vi "ExperimentProgramUI.vi"() -> ()   [LabVIEW 2011]
uses:
  Motors/MotorAxisEnum.ctl
  Motors/MotorPosType.ctl
  Typedefs/XYf.ctl
  Motors/MotorPosFlagsType.ctl
  Typedefs/MeasureConfigOutputMode.ctl
  Typedefs/CmdEnum_UserInterfaceCmd.ctl
  GlobalVariables.vi
panel:
  in  "Run sections util":bool
  in  "Run experiment":bool
  in  "Which motors should the script control?":T1={"Magnet Z"=TRUE, "Magnet rotation"=TRUE, "Camera"={"X"=FALSE, "Y"=FALSE}, "Piezo XY"={"X"=FALSE, "Y"=FALSE}, "Piezo Z"=FALSE, "Coil XY"={"X"=FALSE, "Y"=FALSE}}
  in  "Program.Motor Axis accuracy conditions":T2
  out "Simulated positions":T2[](array[typedef])
  in  "Axis to show in graph":T4[](array[typedef])=[enum."magrot", enum."magrot", enum."magpos"]
  out "Positions according to program":dbl[][](graph)
  in  "Tab Control 2":enum32{"Script", "Paths & Settings"}(tab)
  in  "Test run without experiment":bool
  in  "Script":string="% Initial position\n%move magpos 20; move magrot 0;\n%wait\n\n% Program\n%move magrot 1000 speed 100; wait;\n%move magrot 50 speed 10;\n%move magpos 10 speed 2;wait\n"
  in  "Simulate script":bool
  in  "Save script":bool
  in  "Load script":bool
  in  "Write interval [frames]":i32
  in  "Experiment base path":path
  in  "Experiment name":string
  out "Traces will end up here:":path
  in  "Output mode":T5=enum."Track"
  in  "Image output path":string
  in  "Trace output path":string
  in  "Max frames in memory":i32
  in  "Save traces as binary":bool
  in  "stop":bool
  # "Axis names:\nmagrot:   Magnet rotation\nmagpos:   Magnet Z (vertical) position\npx, py, pz:   Piezo stage\ncamx, camy: Camera motorized stage"
  # "Instructions:\nmove <axis> <position>;\nMove axis to position at current speed\nmove <axis> <position> speed <speed>;\nMove axis to position at specified speed (units/s)\nidle <seconds>;\nDo nothing for specified time\nsection <optional name>;\nStore current framenumber in section file\nstop;\nStop experiment"
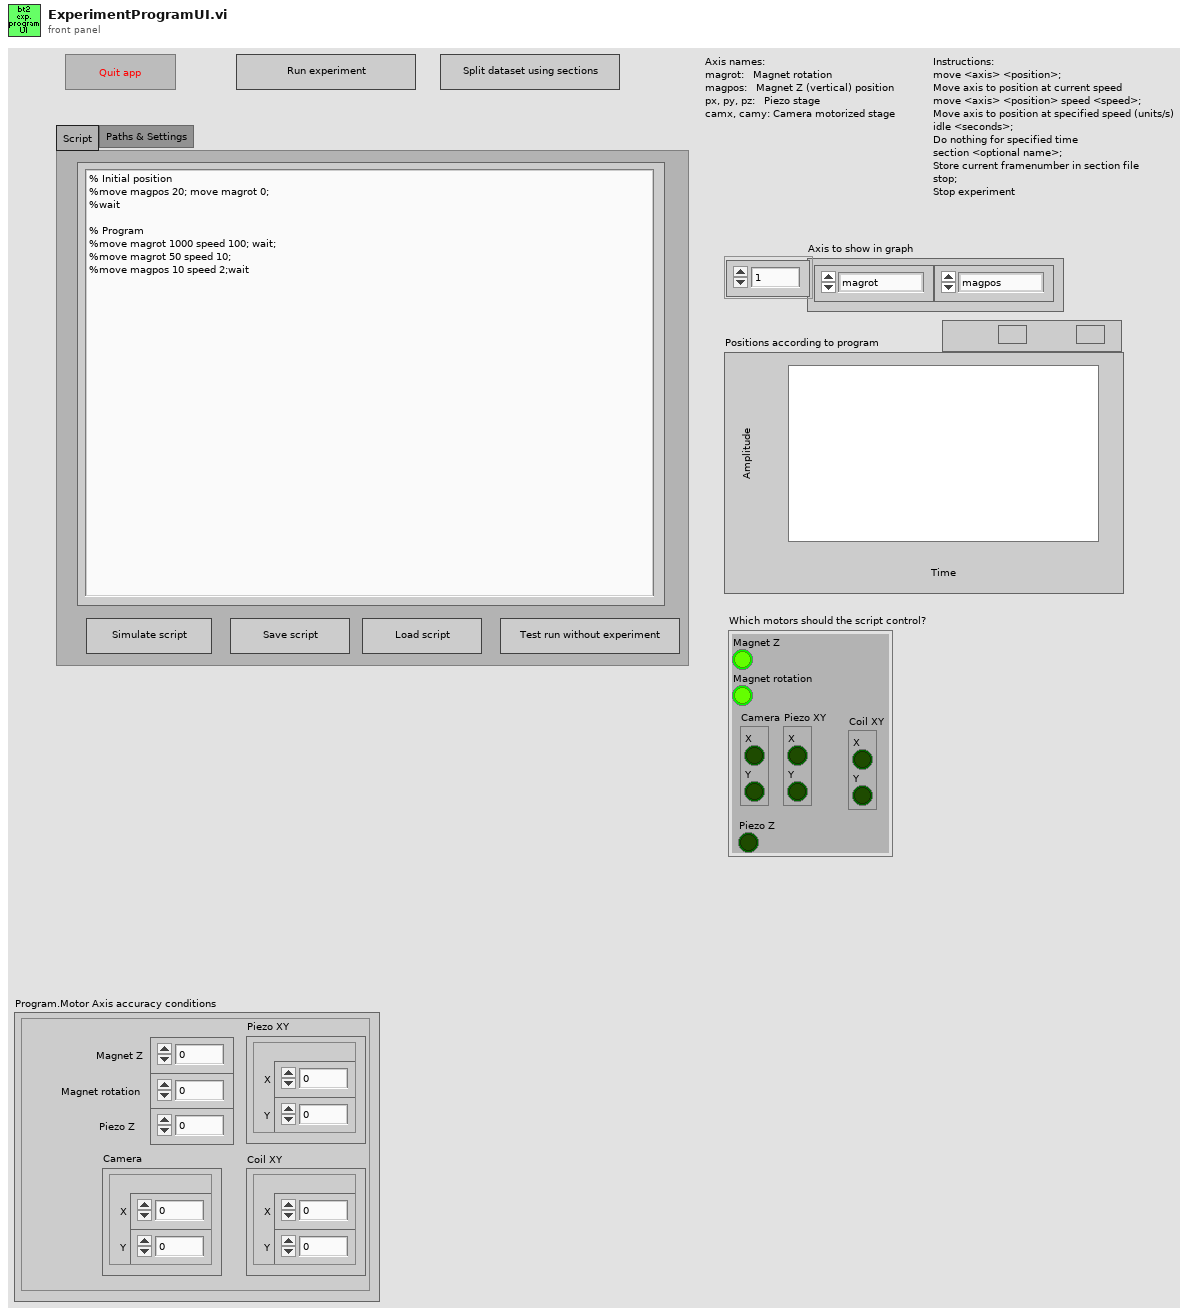
[diagram p1: front panel]
types:
  T1 = typedef "MotorPosFlagsType.ctl" = cluster{"Magnet Z":bool, "Magnet rotation":bool, "Camera":cluster{"X":bool, "Y":bool}, "Piezo XY":cluster{"X":bool, "Y":bool}, "Piezo Z":bool, "Coil XY":cluster{"X":bool, "Y":bool}}
  T2 = typedef "MotorPosType.ctl" = cluster{"Magnet Z":dbl, "Magnet rotation":dbl, "Camera":T3, "Piezo XY":T3, "Piezo Z":dbl, "Coil XY":T3}
  T3 = typedef "XYf.ctl" = cluster{"X":sgl, "Y":sgl}
  T4 = typedef "MotorAxisEnum.ctl" = enum16{"no axis", "magrot", "magpos", "px", "py", "pz", "camx", "camy"}
  T5 = typedef "MeasureConfigOutputMode.ctl" = enum16{"None", "Track", "SaveImages"}
  T6 = cluster{"UpdateGraphEvent":refnum<user-event>, "MeasureConfigUpdated":refnum<user-event>}
  T7 = typedef "QueueListType.ctl" = cluster{"Motor In":refnum<queue>, "User Interface Image View":refnum<queue>, "User Interface Camera Control":refnum<queue>, "User Interface Event Notifier":refnum<notifier>, "Initialized?":bool}
  T8 = typedef "CmdEnum_UserInterfaceCmd.ctl" = enum32{"Idle (Use for default)", "ResultTracesUpdated", "MeasureConfigUpdated", "MeasureEnd", "MeasureStart"}
  T9 = typedef "MeasureConfigType.ctl" = cluster{"Bead locations":cluster{"X":i32, "Y":i32}[], "ROI":i32, "Experiment base path":path, "Image output subdir":string, "Output mode":T5, "Traces output subdir":string, "QTrk Settings":T10, "Tracking Config":T11, "Experiment Name":string, "Program":T14, "ZLUT":sgl[][][], "Camera settings":T17, "Experiment Script":string, "Max frames in memory":i32, "Save traces as binary":bool, "Pixel Calibration Gain Image":string, "Pixel Calibration Offset Image":string, "Use pixel calibration images":bool, "Internal camera settings":string, "Trace write interval":i32}
  T10 = typedef "QTrkSettings.ctl" = cluster{"Image width":i32, "Image height":i32, "Number of threads (CPU based)":i32, "CUDA Device":i32, "COM Background correction factor":sgl, "ZLUT MinRadius":sgl, "ZLUT Radial sample density":sgl, "ZLUT Angular sample density":sgl, "ZLUT ROI Coverage":sgl, "QI Iterations":i32, "QI MinRadius":sgl, "QI Radial sample density":sgl, "QI Angular sample density":sgl, "QI ROI Coverage":sgl, "QI Angular Step \nIteration Factor":sgl, "XCOR Profile Length":i32, "XCOR Profile Width":i32, "XCOR Iterations":i32, "Gaussian 2D Fit Iterations":i32, "Gaussian 2D Sigma (pixels)":sgl, "Downsample":i32}
  T11 = typedef "TrackingConfigType.ctl" = cluster{"Number of steps":i32, "ZLUT stepsize (um)":sgl, "Z correction factor":sgl, "Start piezo Z (um)":sgl, "Pixel size (nm)":sgl, "2D Localization Type":T12, "Z Command (None)":T13, "Z Piezo scale":bool, "ZLUT Building\nimages per frame":i32}
  T12 = typedef "QTrkLocalizationType.ctl" = enum16{"Center-of-Mass", "1D Cross-Correlation", "Quadrant Interpolation", "Gaussian 2D MLE", "QI + ZLUTAlign", "ZLUTAlign", "QI + FourierLUT"}
  T13 = typedef "QTrkZCommandType.ctl" = enum16{"Nothing", "ComputeZ", "BuildRadialZLUT", "BuildImageZLUT", "RadialZLUT+ImageZLUT"}
  T14 = typedef "ExperimentProgramType.ctl" = cluster{"Commands":T15[], "Motor Axis accuracy conditions":T2, "Axis flags":T1}
  T15 = typedef "ExProgCommandType.ctl" = cluster{"cmd":T16, "axis":T4, "value/pos":dbl, "speed":dbl, "name":string}
  T16 = typedef "ExProgCommandEnumType.ctl" = enum16{"wait", "move", "acquire", "idle", "rmove", "when", "section", "stop"}
  T17 = typedef "GenericCameraConfigType.ctl" = cluster{"Framerate (Hz)":i32, "Exposure time (us)":i32, "Image size":cluster{"Width":i32, "Height":i32}, "Number of buffers":i32}
  T18 = typedef "UserInterfaceEventType.ctl" = cluster{"Type":T8}
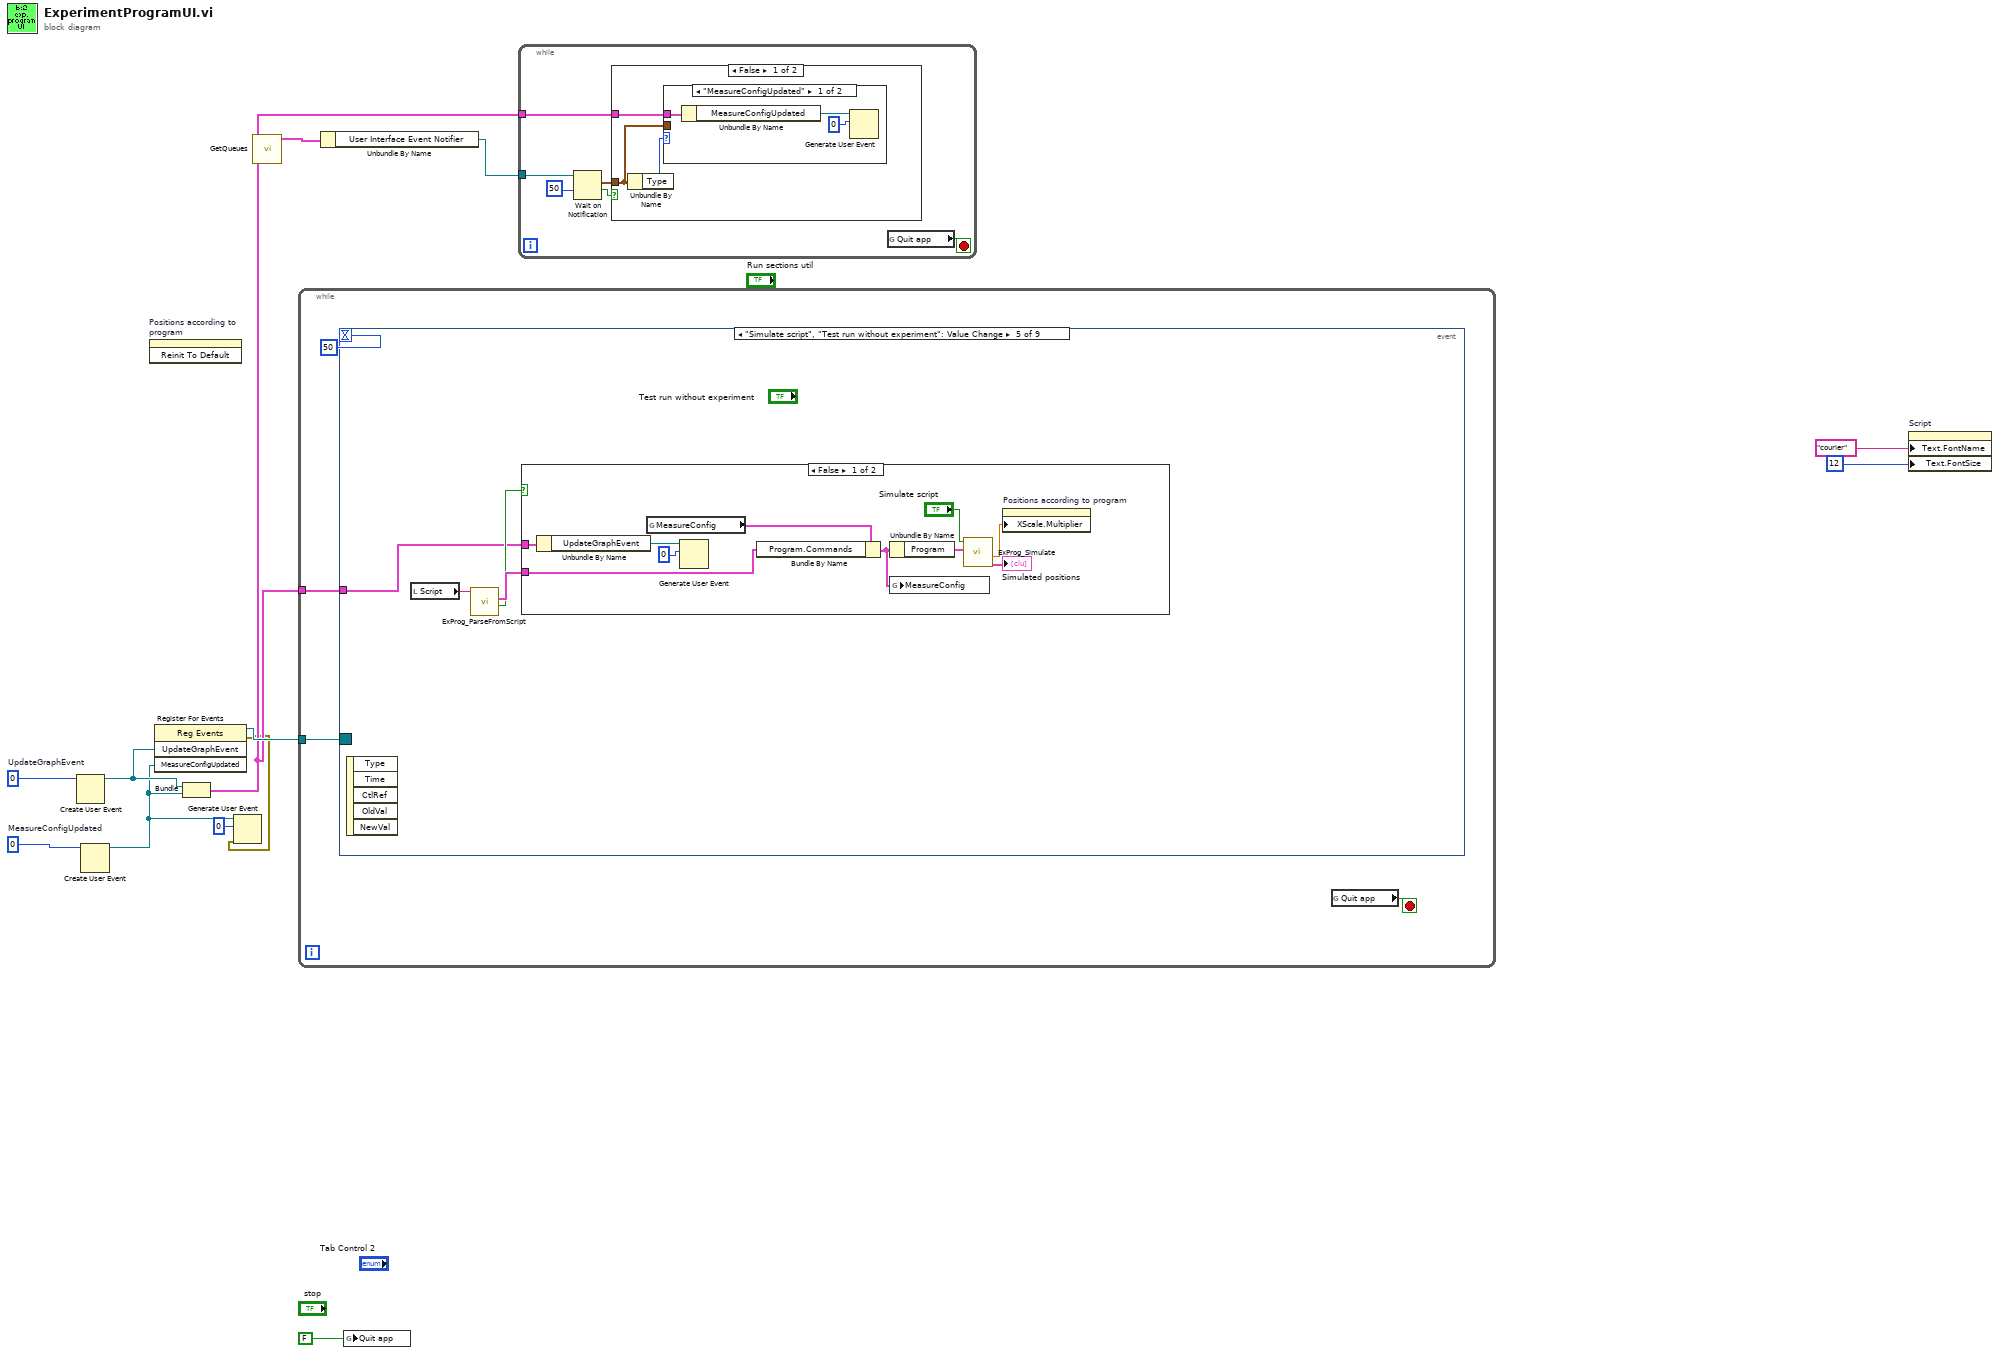
[diagram p0: block diagram]
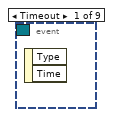
[diagram p4: hidden frame]
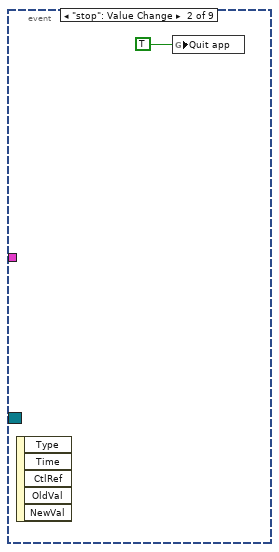
[diagram p5: hidden frame]
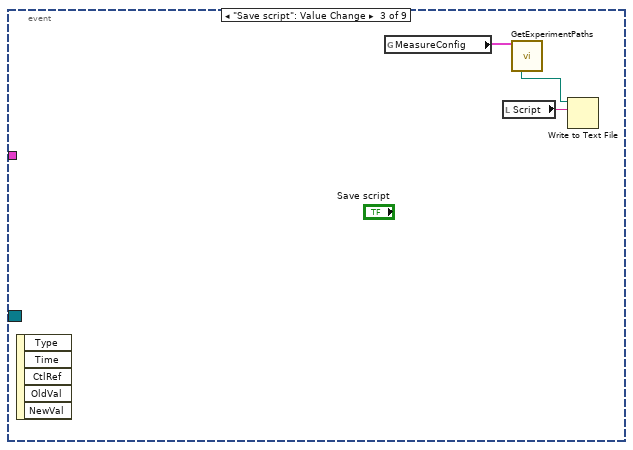
[diagram p6: hidden frame]
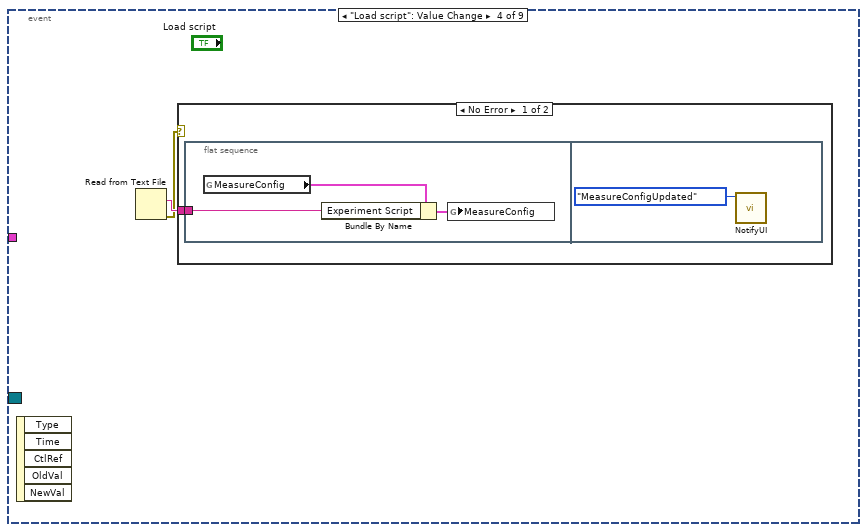
[diagram p7: hidden frame]
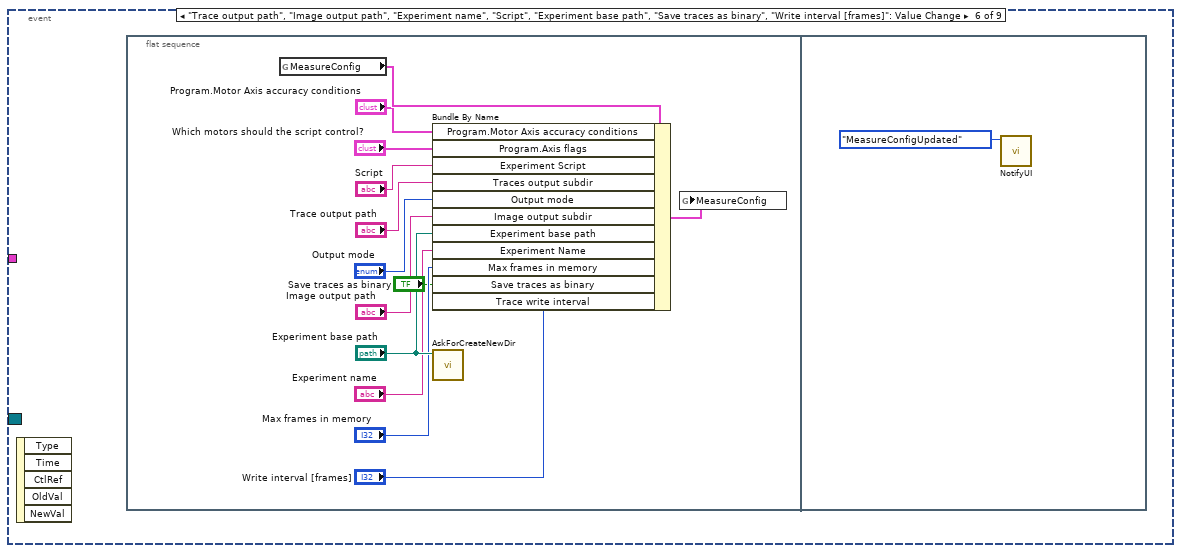
[diagram p10: hidden frame]
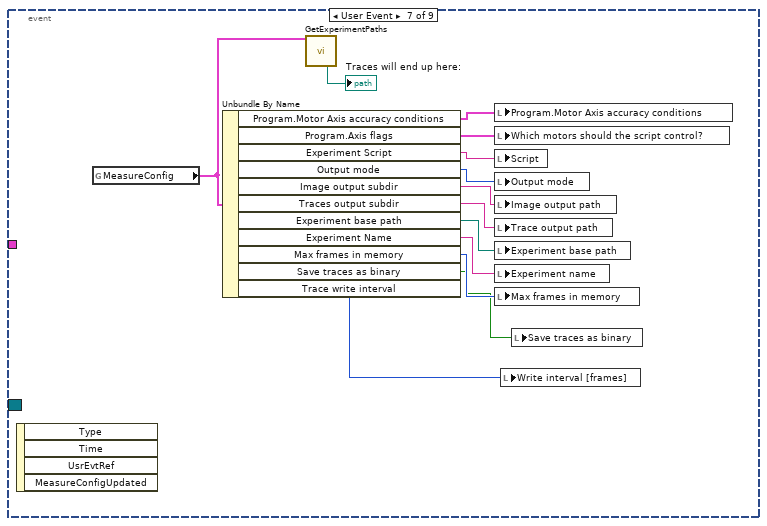
[diagram p11: hidden frame]
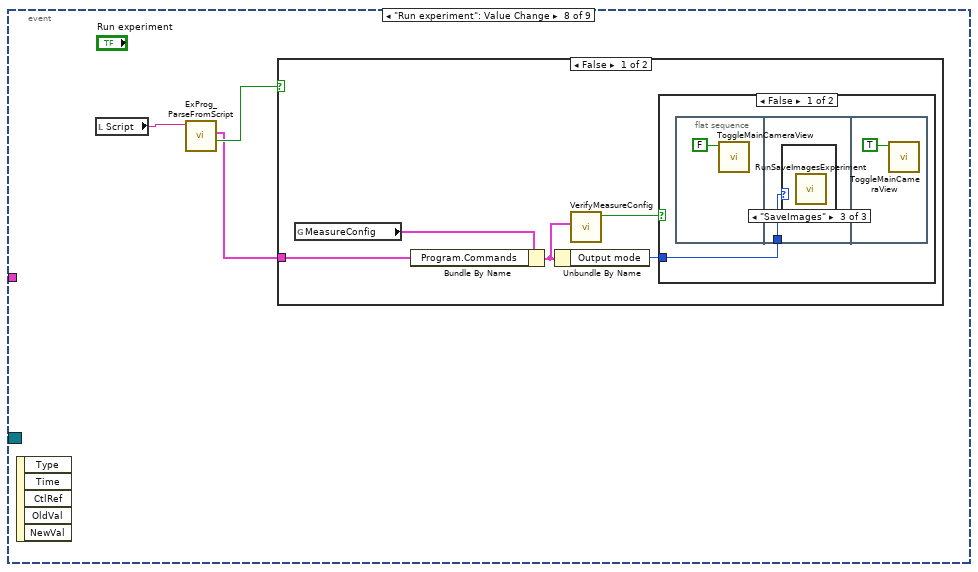
[diagram p12: hidden frame]
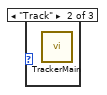
[diagram p14: hidden frame]
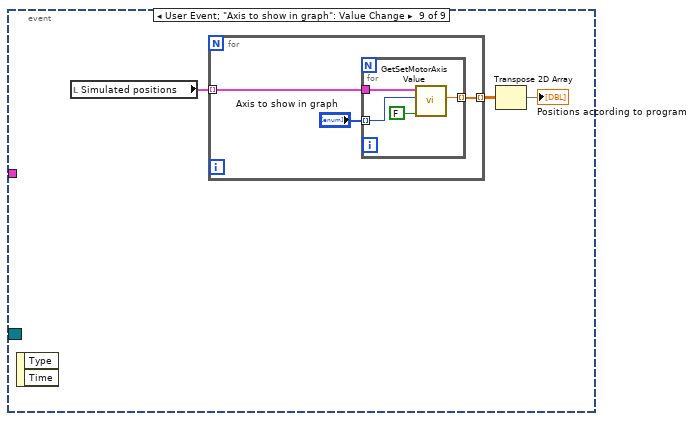
[diagram p17: hidden frame]
diagram:
  w6 = 0  # MeasureConfigUpdated
  w8 = 0  # UpdateGraphEvent
  n1 = Create User Event(user event datatype=w8) -> (user event=w7:refnum<user-event>)  [unwired: 1 in, 1 out]
  n2 = Create User Event(user event datatype=w6) -> (user event=w4:refnum<user-event>)  [unwired: 1 in, 1 out]
  n3 = invoke on="Positions according to program" class="WFGraph (strict)" method="Reinit To Default"() -> ()  [unwired: 3 in, 3 out]
  n4 = register-events(w7, w4) -> (reference out=w9:refnum<event-registration>, error out=w2:errorcluster)  [unwired: 2 in]
  n5 = Bundle("UpdateGraphEvent"=w7, "MeasureConfigUpdated"=w4) -> (w5:T6)  [unwired: 1 in]
  n6 = Generate User Event(user event=w4, event data cluster=0 ("event data"), error in=w2) -> ()  [unwired: 2 out]
  n7 = call "GetQueues.vi"() -> ("Queue List"=w10:T7)  [unwired: 10 in, 1 out]
  n8 = while {
    tunnel: w9 -> [w15]
    tunnel: w5 -> [w14]
    stop <- w17 stop-if-true
    n9 = event shown="[4] \"Simulate script\", \"Test run without experiment\": Value Change" {
      selector: w15 -> [_ _ _ _ _ _ _ _ _]
      dyn-events: _ -> [_ _ _ _ _ _ _ _ _]
      timeout: 50 -> [_ _ _ _ _ _ _ _ _]
      tunnel: w14 -> [_ _ _ _ w30 _ _ _ _]
      event Timeout {
        n10 = event-data() -> ()  [unwired: 1 in, 2 out]
      }
      event "stop": Value Change {
        n11 = event-data() -> ()  [unwired: 1 in, 5 out]
        n12 = global write "GlobalVariables.vi" "Quit app"(TRUE ("Quit app")) -> ()
      }
      event "Save script": Value Change {
        n13 = event-data() -> ()  [unwired: 1 in, 5 out]
        n14 = global read "GlobalVariables.vi" "MeasureConfig"() -> (w21:T9)
        n15 = local read "Script"() -> (w20:string)
        n16 = call "GetExperimentPaths.vi"("MeasureConfig"=w21) -> ("[base]\\[expname]_script.txt"=w19:path)  [unwired: 6 in, 8 out]
        n17 = Write to Text File(file (use dialog)=w19, text=w20) -> ()  [unwired: 2 in, 3 out]
      }
      event "Load script": Value Change {
        n18 = event-data() -> ()  [unwired: 1 in, 5 out]
        n19 = Read from Text File() -> (text=w23:string, error out=w22:errorcluster)  [unwired: 4 in, 2 out]
        n20 = case shown="No Error" w22 {
          tunnel: w23 -> [w24 _]
          frame No Error {
            n21 = flat-sequence {
              tunnel: w24 -> [w25]
              frame #0 {
                n22 = global read "GlobalVariables.vi" "MeasureConfig"() -> (w26:T9)
                n23 = Bundle By Name(cluster=w26, "Experiment Script"=w25) -> (w27:T9)
                n24 = global write "GlobalVariables.vi" "MeasureConfig"(w27) -> ()
              }
              frame #1 {
                n25 = call "NotifyUI.vi"("User Interface Commands"=CmdEnum_UserInterfaceCmd."MeasureConfigUpdated") -> ()  [unwired: 11 in]
              }
            }
          }
          frame Error {
          }
        }
      }
      event "Simulate script", "Test run without experiment": Value Change {
        n26 = event-data() -> ()  [unwired: 1 in, 5 out]
        n27 = local read "Script"() -> (w29:string)
        n28 = call "ExProg_ParseFromScript.vi"("text"=w29) -> ("error?"=w31:bool, "program"=w32:T15[])  [unwired: 9 in]
        n29 = case shown="False" w31 {
          tunnel: w32 -> [w41 _]
          tunnel: w30 -> [w37 _]
          frame False {
            n30 = Unbundle By Name(w37) -> ("UpdateGraphEvent"=w36:refnum<user-event>)
            n31 = global read "GlobalVariables.vi" "MeasureConfig"() -> (w42:T9)
            n32 = Generate User Event(user event=w36, event data cluster=0 ("event data")) -> ()  [unwired: 1 in, 2 out]
            n33 = Bundle By Name(cluster=w42, "Program.Commands"=w41) -> (w40:T9)
            n34 = Unbundle By Name(w40) -> ("Program"=w39:T14)
            n35 = global write "GlobalVariables.vi" "MeasureConfig"(w40) -> ()
            n36 = call "ExProg_Simulate.vi"("Program"=w39, "Simulation?"="Simulate script") -> ("Wanted position list"=→"Simulated positions":T2[], "Used timestep (s)"=w38:sgl)  [unwired: 8 in]
            n37 = property on="Positions according to program" class="WFGraph (strict)"("XScale.Multiplier"=w38) -> ()  [unwired: 2 in, 2 out]
          }
          frame True {
          }
        }
      }
      event "Trace output path", "Image output path", "Experiment name", "Script", "Experiment base path", "Save traces as binary", "Write interval [frames]": Value Change {
        n38 = event-data() -> ()  [unwired: 1 in, 5 out]
        n39 = flat-sequence {
          frame #0 {
            n40 = global read "GlobalVariables.vi" "MeasureConfig"() -> (w55:T9)
            n41 = Bundle By Name(cluster=w55, "Program.Motor Axis accuracy conditions"="Program.Motor Axis accuracy conditions", "Program.Axis flags"="Which motors should the script control?", "Experiment Script"="Script", "Traces output subdir"="Trace output path", "Output mode"="Output mode", "Image output subdir"="Image output path", "Experiment base path"="Experiment base path", "Experiment Name"="Experiment name", "Max frames in memory"="Max frames in memory", "Save traces as binary"="Save traces as binary", "Trace write interval"="Write interval [frames]") -> (w54:T9)
            n42 = call "AskForCreateNewDir.vi"("Experiment base path"="Experiment base path") -> ()  [unwired: 11 in]
            n43 = global write "GlobalVariables.vi" "MeasureConfig"(w54) -> ()
          }
          frame #1 {
            n44 = call "NotifyUI.vi"("User Interface Commands"=CmdEnum_UserInterfaceCmd."MeasureConfigUpdated") -> ()  [unwired: 11 in]
          }
        }
      }
      event User Event {
        n45 = event-data() -> ()  [unwired: 1 in, 4 out]
        n46 = global read "GlobalVariables.vi" "MeasureConfig"() -> (w63:T9)
        n47 = Unbundle By Name(w63) -> ("Program.Motor Axis accuracy conditions"=w69:T2, "Program.Axis flags"=w68:T1, "Experiment Script"=w67:string, "Output mode"=w66:T5, "Image output subdir"=w65:string, "Traces output subdir"=w64:string, "Experiment base path"=w61:path, "Experiment Name"=w60:string, "Max frames in memory"=w59:i32, "Save traces as binary"=w58:bool, "Trace write interval"=w57:i32)
        n48 = call "GetExperimentPaths.vi"("MeasureConfig"=w63) -> ("[base]\\traces\\[expname].txt/bin"=→"Traces will end up here:":path)  [unwired: 6 in, 8 out]
        n49 = local write "Program.Motor Axis accuracy conditions"(w69) -> ()
        n50 = local write "Which motors should the script control?"(w68) -> ()
        n51 = local write "Script"(w67) -> ()
        n52 = local write "Output mode"(w66) -> ()
        n53 = local write "Image output path"(w65) -> ()
        n54 = local write "Trace output path"(w64) -> ()
        n55 = local write "Experiment base path"(w61) -> ()
        n56 = local write "Experiment name"(w60) -> ()
        n57 = local write "Max frames in memory"(w59) -> ()
        n58 = local write "Write interval [frames]"(w57) -> ()
        n59 = local write "Save traces as binary"(w58) -> ()
      }
      event "Run experiment": Value Change {
        n60 = event-data() -> ()  [unwired: 1 in, 5 out]
        n61 = local read "Script"() -> (w72:string)
        n62 = call "ExProg_ParseFromScript.vi"("text"=w72) -> ("error?"=w71:bool, "program"=w70:T15[])  [unwired: 9 in]
        n63 = case shown="False" w71 {
          tunnel: w70 -> [w74 _]
          frame False {
            n64 = global read "GlobalVariables.vi" "MeasureConfig"() -> (w76:T9)
            n65 = Bundle By Name(cluster=w76, "Program.Commands"=w74) -> (w75:T9)
            n66 = Unbundle By Name(w75) -> ("Output mode"=w77:T5)
            n67 = call "VerifyMeasureConfig.vi"("MeasureConfig"=w75) -> ("Cancel button pressed?"=w73:bool)  [unwired: 10 in]
            n68 = case shown="False" w73 {
              tunnel: w77 -> [w78 _]
              frame False {
                n69 = flat-sequence {
                  tunnel: w78 -> [w80]
                  frame #0 {
                    n70 = call "ToggleMainCameraView.vi"("Enable? (T)"=FALSE) -> ()  [unwired: 11 in]
                  }
                  frame #1 {
                    n71 = case shown="\"SaveImages\"" w80 {
                      frame "None", Default {
                      }
                      frame "Track" {
                        n72 = call "TrackerMain.vi"() -> ()  [unwired: 11 in, 1 out]
                      }
                      frame "SaveImages" {
                        n73 = call "RunSaveImagesExperiment.vi"() -> ()  [unwired: 12 in]
                      }
                    }
                  }
                  frame #2 {
                    n74 = call "ToggleMainCameraView.vi"("Enable? (T)"=TRUE) -> ()  [unwired: 11 in]
                  }
                }
              }
              frame True {
              }
            }
          }
          frame True {
          }
        }
      }
      event User Event; "Axis to show in graph": Value Change {
        n75 = event-data() -> ()  [unwired: 1 in, 2 out]
        n76 = local read "Simulated positions"() -> (w84:T2[])
        n77 = for {
          tunnel: w84 -> [w86] mode=indexing
          tunnel: [w85] -> w83 mode=indexing
          n78 = for {
            tunnel: "Axis to show in graph" -> [w90] mode=indexing
            tunnel: w86 -> [w91]
            tunnel: [w88] -> w85 mode=indexing
            n79 = call "GetSetMotorAxisValue.vi"("set? (T)"=FALSE, "axis"=w90, "Motorpos in"=w91) -> ("pos (out)"=w88:dbl)  [unwired: 7 in, 1 out]
          }
        }
        n80 = Transpose 2D Array(2D array=w83) -> (transposed array=→"Positions according to program":dbl[][])
      }
    }
    n81 = global read "GlobalVariables.vi" "Quit app"() -> (w17:bool)
  }
  n82 = Unbundle By Name(w10) -> ("User Interface Event Notifier"=w1:refnum<notifier>)
  n83 = global write "GlobalVariables.vi" "Quit app"(FALSE ("Quit app")) -> ()
  n84 = while {
    tunnel: w5 -> [w96]
    tunnel: w1 -> [w95]
    stop <- w97 stop-if-true
    n85 = Wait on Notification(notifier=w95, timeout in ms (-1)=50) -> (notification=w94:T18, timed out?=w92:bool)  [unwired: 2 in, 2 out]
    n86 = case shown="False" w92 {
      tunnel: w96 -> [w100 _]
      tunnel: w94 -> [w99 _]
      frame False {
        n87 = Unbundle By Name(w99) -> ("Type"=w98:T8)
        n88 = case shown="\"MeasureConfigUpdated\"" w98 {
          tunnel: w99 -> [_ _]
          tunnel: w100 -> [w103 _]
          frame "MeasureConfigUpdated" {
            n89 = Unbundle By Name(w103) -> ("MeasureConfigUpdated"=w102:refnum<user-event>)
            n90 = Generate User Event(user event=w102, event data cluster=0 ("event data")) -> ()  [unwired: 1 in, 2 out]
          }
          frame "Idle (Use for default)", Default {
          }
        }
      }
      frame True {
      }
    }
    n91 = global read "GlobalVariables.vi" "Quit app"() -> (w97:bool)
  }
  n92 = property on="Script" class="Str"("Text.FontName"="courier" ("Text.Font:Name"), "Text.FontSize"=u32 12 ("Text.Font:Size")) -> ()  [unwired: 2 in, 2 out]
